vi "Enable Timer.vi"(8 "error in (no error)":errorcluster, 9 "Enable Timer (Disable)":bool, 10 "Channel (1:CH1)":u16(ring)=1 items=["CH1"=1, "CH2"=2], 11 "VISA resource name":refnum<visa-resource-name>) -> (0 "error out":errorcluster, 3 "VISA resource name out":refnum<visa-resource-name>)   [LabVIEW 2015, in "Siglent SPD3000 Series.lvlib"]
doc: "Turns on or off the timer function of selected channel.\n\n<B>Note:</B>\nThis VI is invalid for the SPD3303C models."
uses:
  <instrlib>/Siglent SPD3000 Series/Siglent SPD3000 Series.lvlib
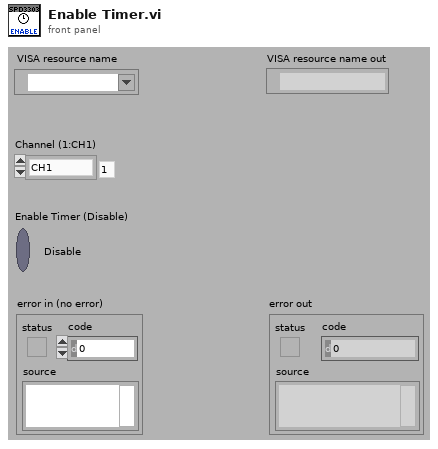
[diagram p1: front panel]
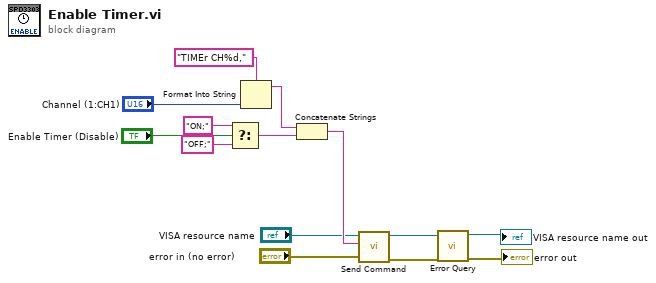
[diagram p0: block diagram]
diagram:
  n1 = Select(t="ON;" ("写入缓冲区"), s="Enable Timer (Disable)", f="OFF;" ("写入缓冲区")) -> (s? t:f=w7:string)
  n2 = Format Into String(format string="TIMEr CH%d," ("写入缓冲区"), "Channel (1:CH1)") -> (resulting string=w8:string)  [unwired: 2 in, 1 out]
  n3 = Concatenate Strings(w8, w7) -> (w6:string)
  n4 = call <instrlib>:"Send Command.vi"("error in (no error)"="error in (no error)", "Write Buffer (\"\")"=w6, "VISA resource name"="VISA resource name") -> ("error out"=w11:errorcluster, "VISA resource name out"=w12:refnum<visa-resource-name>)  [unwired: 7 in]
  n5 = call <instrlib>:"Error Query.vi"("error in (no error)"=w11, "VISA resource name"=w12) -> ("error out"=→"error out":errorcluster, "VISA resource name out"=→"VISA resource name out":refnum<visa-resource-name>)  [unwired: 6 in, 2 out]
